vi "SIM921_Queue_Commands.vi"(1 "SIM921-Control":T1, 3 "SIM Queue":refnum<queue>) -> (0 "SIM921-Control new status":T1)   [LabVIEW 2019]
uses:
  SIM921/SIM921_control_cluster.ctl
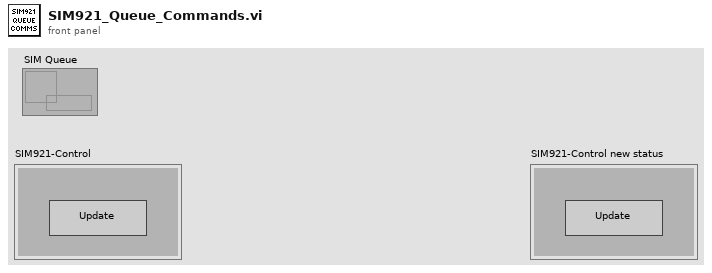
[diagram p1: front panel]
types:
  T1 = typedef "SIM921_control_cluster.ctl" = cluster{"Update":bool}
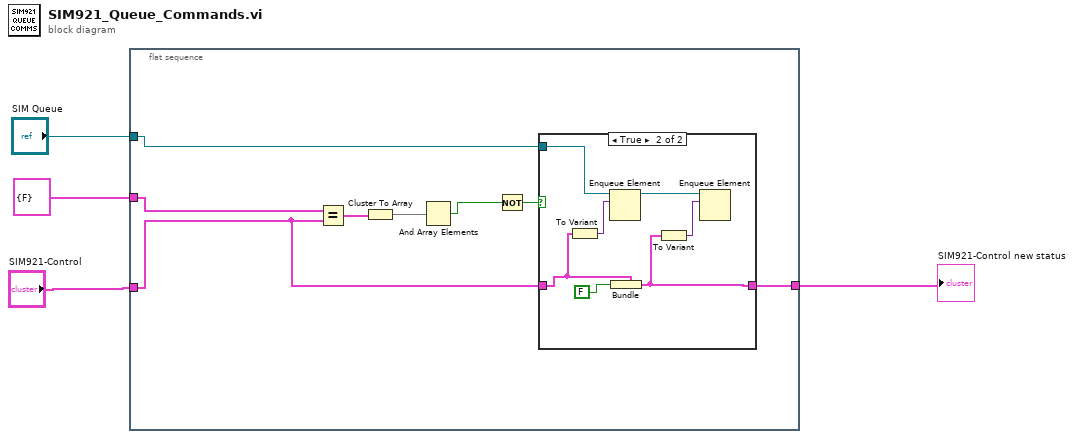
[diagram p0: block diagram]
diagram:
  n1 = flat-sequence {
    tunnel: T1 {"Update"=FALSE} ("SIM921-Control") -> [w12]
    tunnel: "SIM921-Control" -> [w6]
    tunnel: "SIM Queue" -> [w7]
    tunnel: [w5] -> w1
    frame #0 {
      n2 = Equal?(x=w12, y=w6) -> (x = y?=w11:T1)
      n3 = Cluster To Array(cluster=w11) -> (array=w10:bool[])
      n4 = And Array Elements(Boolean array=w10) -> (logical AND=w9:bool)
      n5 = Not(x=w9) -> (.not. x?=w8:bool)
      n6 = case shown="True" w8 {
        tunnel: w7 -> [_ w20]
        tunnel: w6 -> [w13 w16]
        tunnel: [w13 w14] -> w5
        frame False {
        }
        frame True {
          n7 = To Variant(anything=w16) -> (Variant=w17:variant)
          n8 = Enqueue Element(queue=w20, element=w17) -> (queue out=w19:refnum<queue>)  [unwired: 2 in, 2 out]
          n9 = Bundle(cluster=w16, "Update"=FALSE) -> (w14:T1)
          n10 = To Variant(anything=w14) -> (Variant=w15:variant)
          n11 = Enqueue Element(queue=w19, element=w15) -> ()  [unwired: 2 in, 3 out]
        }
      }
    }
  }
  "SIM921-Control new status" <- w1
